vi "Parse Core.vi"(0 "SG SC2250 Path in":refnum<class "SG SC2250 Path.lvclass">, 5 "Config Row":string[](array[string]), 11 "error in (no error)":errorcluster) -> (4 "SG SC2250 Path out":refnum<class "SG SC2250 Path.lvclass">, 15 "error out":errorcluster)   [LabVIEW 2023, in "RFFixtureCharact.RFPM.lvlib" / "SG SC2250 Path.lvclass"]
uses:
  SG SC2250 Path.lvclass
  C:/srd-semi-rfcal-software/AuxTools/STSRFFixtureCharactUtility/Source/Code Modules/Common/Base Classes/Path/Path.lvclass
  Charact Result Accessor/Scalar/Scalar Charact Result Accessor.lvclass
  C:/srd-semi-rfcal-software/AuxTools/STSRFFixtureCharactUtility/Source/Code Modules/Fixture/RFPM/Charact Result Accessor/Base/Charact Result Accessor.lvclass
  C:/srd-semi-rfcal-software/AuxTools/STSRFFixtureCharactUtility/Source/Code Modules/Common/Result Accessor/Result Accessor.lvclass
  SG SC2250 Path.lvclass/SG SC2250 Path.ctl
  Common/Base Classes/Path/Path.lvclass/Path.ctl
  Properties/Write Cal Tone Source.vi
  Common/Base Classes/Path/Properties/Read Date.vi
  Common/Base Classes/Path/Properties/Read Interval.vi
  SG Path/SG 18GHz Path.lvclass
  Common/RFCalAndFixtureCharact.Common.lvlib
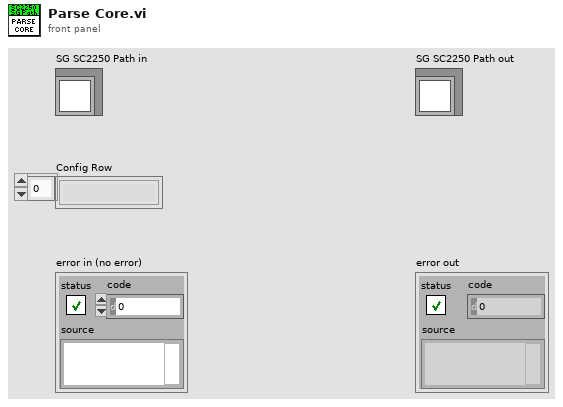
[diagram p1: front panel]
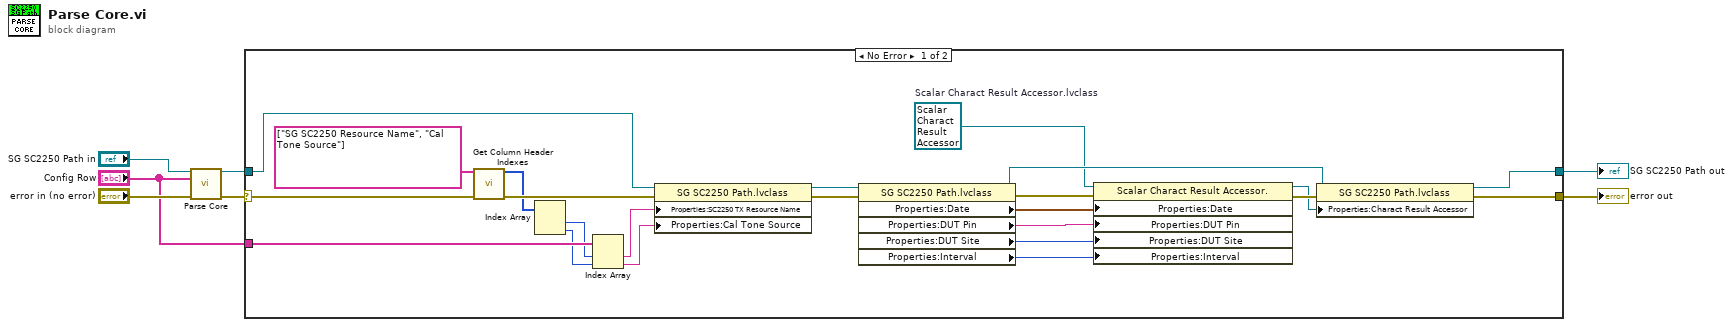
[diagram p0: block diagram]
diagram:
  n1 = call-parent "Parse Core.vi"("SG Path in"="SG SC2250 Path in", "Config Row"="Config Row", "error in"="error in (no error)") -> ("SG Path out"=w2:refnum<class "SG SC2250 Path.lvclass">, "error out"=w1:errorcluster)  [unwired: 11 in]
  n2 = case shown="No Error" w1 {
    selector: w1 -> [w22 w32]
    tunnel: [w10 w32] -> w7
    tunnel: [w9 w31] -> w6
    tunnel: "Config Row" -> [w30 _]
    tunnel: w2 -> [w21 w31]
    frame No Error {
      w12 = refnum<class "Scalar Charact Result Accessor.lvclass"> refnum  # Scalar Charact Result Accessor.lvclass
      n3 = call "Get Column Header Indexes.vi"("Column Header Names"=string[] ["SG SC2250 Resource Name", "Cal Tone Source"], "error in"=w22) -> ("Column Header Indices"=w25:i32[], "error out"=w27:errorcluster)  [unwired: 11 in, 1 out]
      n4 = Index Array(array=w25) -> (element #1=w24:i32, element #2=w23:i32)  [unwired: 2 in]
      n5 = Index Array(array=w30, index #1=w24, index #2=w23) -> (element #1=w29:string, element #2=w28:string)
      n6 = property class="SG SC2250 Path.lvclass"(reference=w21, error in=w27, "Properties:SC2250 TX Resource Name"=w29, "Properties:Cal Tone Source"=w28) -> (reference out=w11:refnum<class "SG SC2250 Path.lvclass">, error out=w8:errorcluster)
      n7 = property class="SG SC2250 Path.lvclass"(reference=w11, error in=w8) -> (reference out=w14:refnum<class "SG SC2250 Path.lvclass">, error out=w19:errorcluster, "Properties:Date"=w18:timestamp, "Properties:DUT Pin"=w17:string, "Properties:DUT Site"=w16:i32, "Properties:Interval"=w15:i32)
      n8 = property class="Scalar Charact Result Accessor."(reference=w12, error in=w19, "Properties:Date"=w18, "Properties:DUT Pin"=w17, "Properties:DUT Site"=w16, "Properties:Interval"=w15) -> (reference out=w13:refnum<class "Scalar Charact Result Accessor.lvclass">, error out=w20:errorcluster)
      n9 = property class="SG SC2250 Path.lvclass"(reference=w14, error in=w20, "Properties:Charact Result Accessor"=w13) -> (reference out=w9:refnum<class "SG SC2250 Path.lvclass">, error out=w10:errorcluster)
    }
    frame Error {
    }
  }
  "error out" <- w7
  "SG SC2250 Path out" <- w6
